vi "Test_Hysteresis_max-LAPTOP-A1ILEVN9.vi"() -> ()   [LabVIEW 2022 SP3]
panel:
  in  "type":enum16{"percentage", "level"}(ring)
  in  "stop":bool
  out "Deviation":bool
  in  "Max":dbl=26.0 format="%#_13g"
  in  "H":dbl=22.0 format="%#_13g"
  in  "input (-)":dbl
  in  "input(+)":dbl
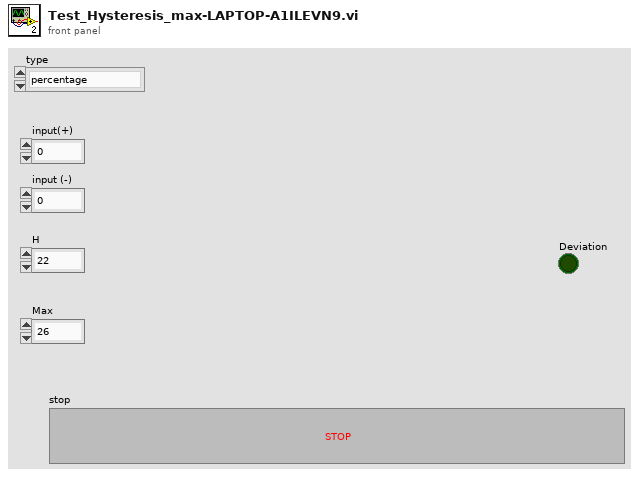
[diagram p1: front panel]
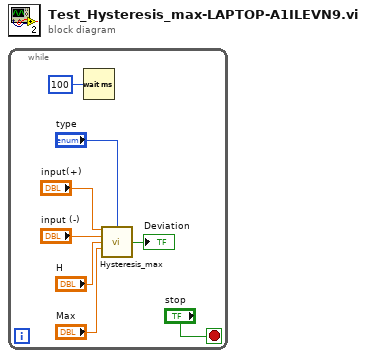
[diagram p0: block diagram]
diagram:
  n1 = while {
    stop <- "stop" stop-if-true
    n2 = Wait (ms)(milliseconds to wait=u32 100) -> ()  [unwired: 1 out]
    n3 = call "Hysteresis_max.vi"("input(+)"="input(+)", "type"="type", "input (-)"="input (-)", "H"="H", "Max"="Max") -> ("Deviation"=→"Deviation":bool)  [unwired: 9 in, 1 out]
  }
